vi "OphirMeasure.vi"(4 "error in (no error)":errorcluster, 5 "Samples":i32, 6 "wavelength":i32, 7 "OphirRef In":T1) -> (0 "error out":errorcluster, 1 "mean":dbl format="%.6g", 2 "median":dbl format="%.6g", 3 "OphirRef Out":T1)   [LabVIEW 2012]
uses:
  TypeDefs/OphirRef.ctl
  <vilib>/Analysis/baseanly.llb/Mean (DBL).vi
  <vilib>/Analysis/NI_AALBase.lvlib
panel:
  out "Array":dbl[](array[numeric])
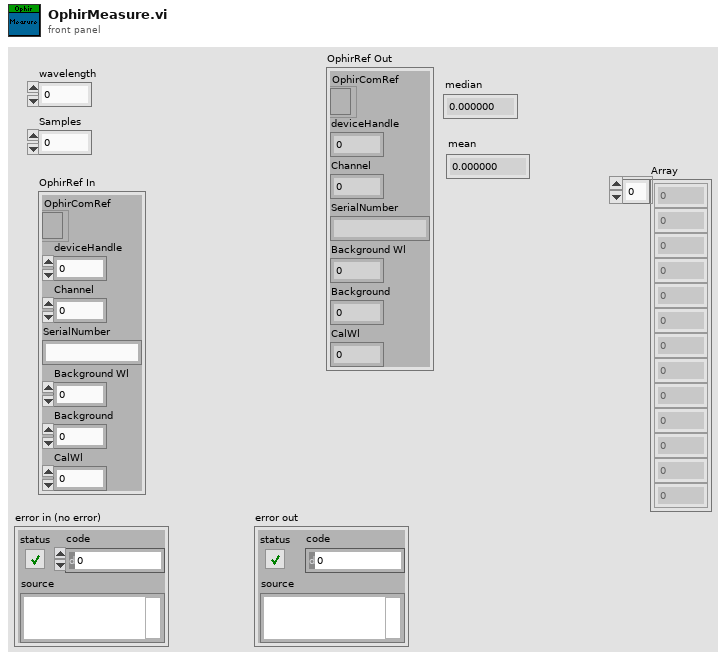
[diagram p1: front panel]
types:
  T1 = typedef "OphirRef.ctl" = cluster{"OphirComRef":refnum<k7>, "deviceHandle":i32, "Channel":i32, "SerialNumber":string, "Background Wl":dbl, "Background":dbl, "CalWl":dbl}
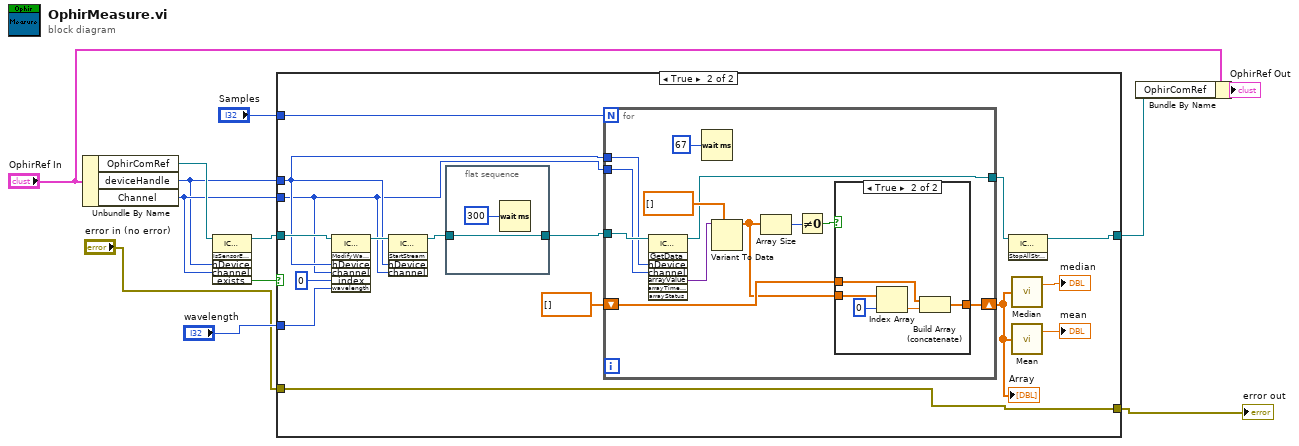
[diagram p0: block diagram]
diagram:
  n1 = Unbundle By Name("OphirRef In") -> ("OphirComRef"=w12:refnum<k7>, "deviceHandle"=w8:i32, "Channel"=w9:i32)
  n2 = invoke class="ICoLMMeasurement2" method="IsSensorExists"(reference=w12, "hDevice"=w8, "channel"=w9) -> (reference out=w10:refnum<k7>, "exists"=w11:bool)  [unwired: 3 in, 4 out]
  n3 = case shown="True" w11 {
    tunnel: w10 -> [w14 w30]
    tunnel: "error in (no error)" -> [w13 w16]
    tunnel: w9 -> [_ w23]
    tunnel: w8 -> [_ w24]
    tunnel: "wavelength" -> [_ w28]
    tunnel: "Samples" -> [_ w26]
    tunnel: [w14 w17] -> w4
    tunnel: [w13 w16] -> w1
    frame False {
    }
    frame True {
      n4 = invoke class="ICoLMMeasurement2" method="ModifyWavelength"(reference=w30, "hDevice"=w24, "channel"=w23, "index"=0, "wavelength"=w28) -> (reference out=w27:refnum<k7>)  [unwired: 2 in, 6 out]
      n5 = invoke on="Invoke Node" class="ICoLMMeasurement2" method="StartStream"(reference=w27, "hDevice"=w24, "channel"=w23) -> (reference out=w15:refnum<k7>)  [unwired: 2 in, 4 out]
      n6 = flat-sequence {
        tunnel: w15 -> [w49]
        tunnel: [w49] -> w25
        frame #0 {
          n7 = Wait (ms)(milliseconds to wait=u32 300) -> ()  [unwired: 1 out]
        }
      }
      n8 = for {
        N: w26 -> [_]
        tunnel: w25 -> [w42]
        tunnel: w24 -> [w41]
        tunnel: w23 -> [w40]
        shift-right: [w34] -> w19
        shift-left: dbl[] [] -> [w36]
        tunnel: [w32] -> w18
        n9 = invoke class="ICoLMMeasurement2" method="GetData"(reference=w42, "hDevice"=w41, "channel"=w40) -> (reference out=w32:refnum<k7>, "arrayValue"=w31:variant)  [unwired: 5 in, 6 out]
        n10 = Wait (ms)(milliseconds to wait=u32 67) -> ()  [unwired: 1 out]
        n11 = Variant To Data(type=dbl[] [], Variant=w31) -> (data=w35:dbl[])  [unwired: 1 in, 1 out]
        n12 = Array Size(array=w35) -> (size(s)=w38:i32)
        n13 = Not Equal To 0?(x=w38) -> (x != 0?=w37:bool)
        n14 = case shown="True" w37 {
          tunnel: w36 -> [w43 w48]
          tunnel: w35 -> [_ w47]
          tunnel: [w43 w44] -> w34
          frame False {
          }
          frame True {
            n15 = Index Array(array=w47, index=0) -> (element=w45:dbl)
            n16 = Build Array (concatenate)(w48, w45) -> (w44:dbl[])
          }
        }
      }
      "Array" <- w19
      n17 = invoke class="ICoLMMeasurement2" method="StopAllStreams"(reference=w18) -> (reference out=w17:refnum<k7>)  [unwired: 2 in, 2 out]
      n18 = call <vilib>:"Median.vi"("X"=w19) -> ("median"=→"median":dbl)  [unwired: 1 out]
      n19 = call-poly <vilib>:"Mean.vi"("X"=w19) -> ("mean"=→"mean":dbl)  [unwired: 1 out]
    }
  }
  "error out" <- w1
  n20 = Bundle By Name(cluster="OphirRef In", "OphirComRef"=w4) -> (→"OphirRef Out":T1)
